vi "ns timing to us timing.vi"(3 "ns timing in":T1) -> (5 "us timing out":T1)   [LabVIEW 2021, in "CIFCoreWrapper.lvlib"]
uses:
  CIFCoreWrapper.lvlib
  Common/Typedef/Timing Stats Base.ctl
  Common/CIFCoreCommon.lvlib
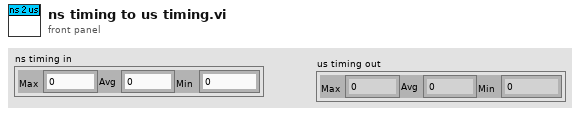
[diagram p1: front panel]
types:
  T1 = typedef "CIFCoreCommon.lvlib/Timing Stats Base.ctl" = cluster{"Max":i64, "Avg":dbl, "Min":i64}
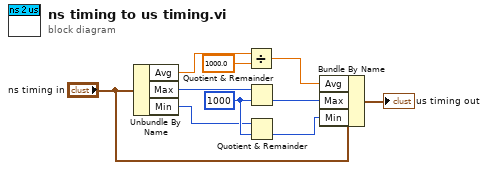
[diagram p0: block diagram]
diagram:
  w6 = i64 1000 ("y")
  n1 = Unbundle By Name("ns timing in") -> ("Avg"=w4:dbl, "Max"=w2:i64, "Min"=w3:i64)
  n2 = Divide(x=w4, y=1000.0) -> (x/y=w8:dbl)
  n3 = Quotient & Remainder(x=w2, y=w6) -> (floor(x/y)=w9:i64)  [unwired: 1 out]
  n4 = Quotient & Remainder(x=w3, y=w6) -> (floor(x/y)=w10:i64)  [unwired: 1 out]
  n5 = Bundle By Name(cluster="ns timing in", "Avg"=w8, "Max"=w9, "Min"=w10) -> (→"us timing out":T1)
